vi "GUI_Bella_Laser.vi"() -> ()   [LabVIEW 2013]
uses:
  shared programs/GUI_Template/GUI_master/tcp_new_data_event.ctl
  shared programs/GUI_Template/GUI_master/tcp new data cluster.ctl
panel:
  out "XY Graph 8":cluster{dbl[], dbl[]}[](graph)
  out "XY Graph 7":cluster{dbl[], dbl[]}[](graph)
  in  "GUIdevice 4":string="LB_EnergyMeter_2"
  in  "GUIdevice 3":string="LB_EnergyMeter_1"
  in  "GUIdevice 2":string="RegenSpectrometer"
  out "FWHM::2":dbl caption="Regen FWHM" min=0.0 max=10000.0
  out "XY Graph 6":cluster{dbl[], dbl[]}[](graph)
  out "Thales.Spectrum_XPW_FWHM::1":dbl caption="Amp2 FWHM" min=-999.0 max=999999999.0
  out "Thales.Spectrum_Amp3_FWHM::1":dbl caption="Amp3 FWHM" min=-999.0 max=999999999.0
  out "Thales.Spectrum_Booster_FWHM::1":dbl caption="Booster FWHM" min=-999.0 max=999999999.0
  out "Thales.Spectrum_Preamp_FWHM::1":dbl caption="Amp1 FWHM" min=-999.0 max=999999999.0
  out "Thales.Spectrum_Regen_FWHM::1":dbl caption="Osc FWHM" min=-999.0 max=999999999.0
  out "XY Graph 5":cluster{dbl[], dbl[]}[](graph)
  in  "Clear":bool
  in  "GUIdevice 1":string="BellaTHALESsveECS"
  out "Reading.Channel 2::4":dbl caption="Amp3 (J)" min=0.0 max=0.0 format="%#.3f"
  out "Reading.Channel 2::3":dbl caption="Amp1 (mJ)" min=0.0 max=0.0
  out "Reading.Channel 1::4":dbl caption="Amp2 (J)" min=0.0 max=0.0 format="%#.3f"
  out "Reading.Channel 1::3":dbl caption="Preamp (mJ)" min=0.0 max=0.0
  out "tcp data event":T1
  in  "stop":bool
  out "error IO 2":errorcluster
  # "BELLA LASER STATS"
  # "Target"
  # "Target"
  # "Target"
  # "Target"
  # "Target"
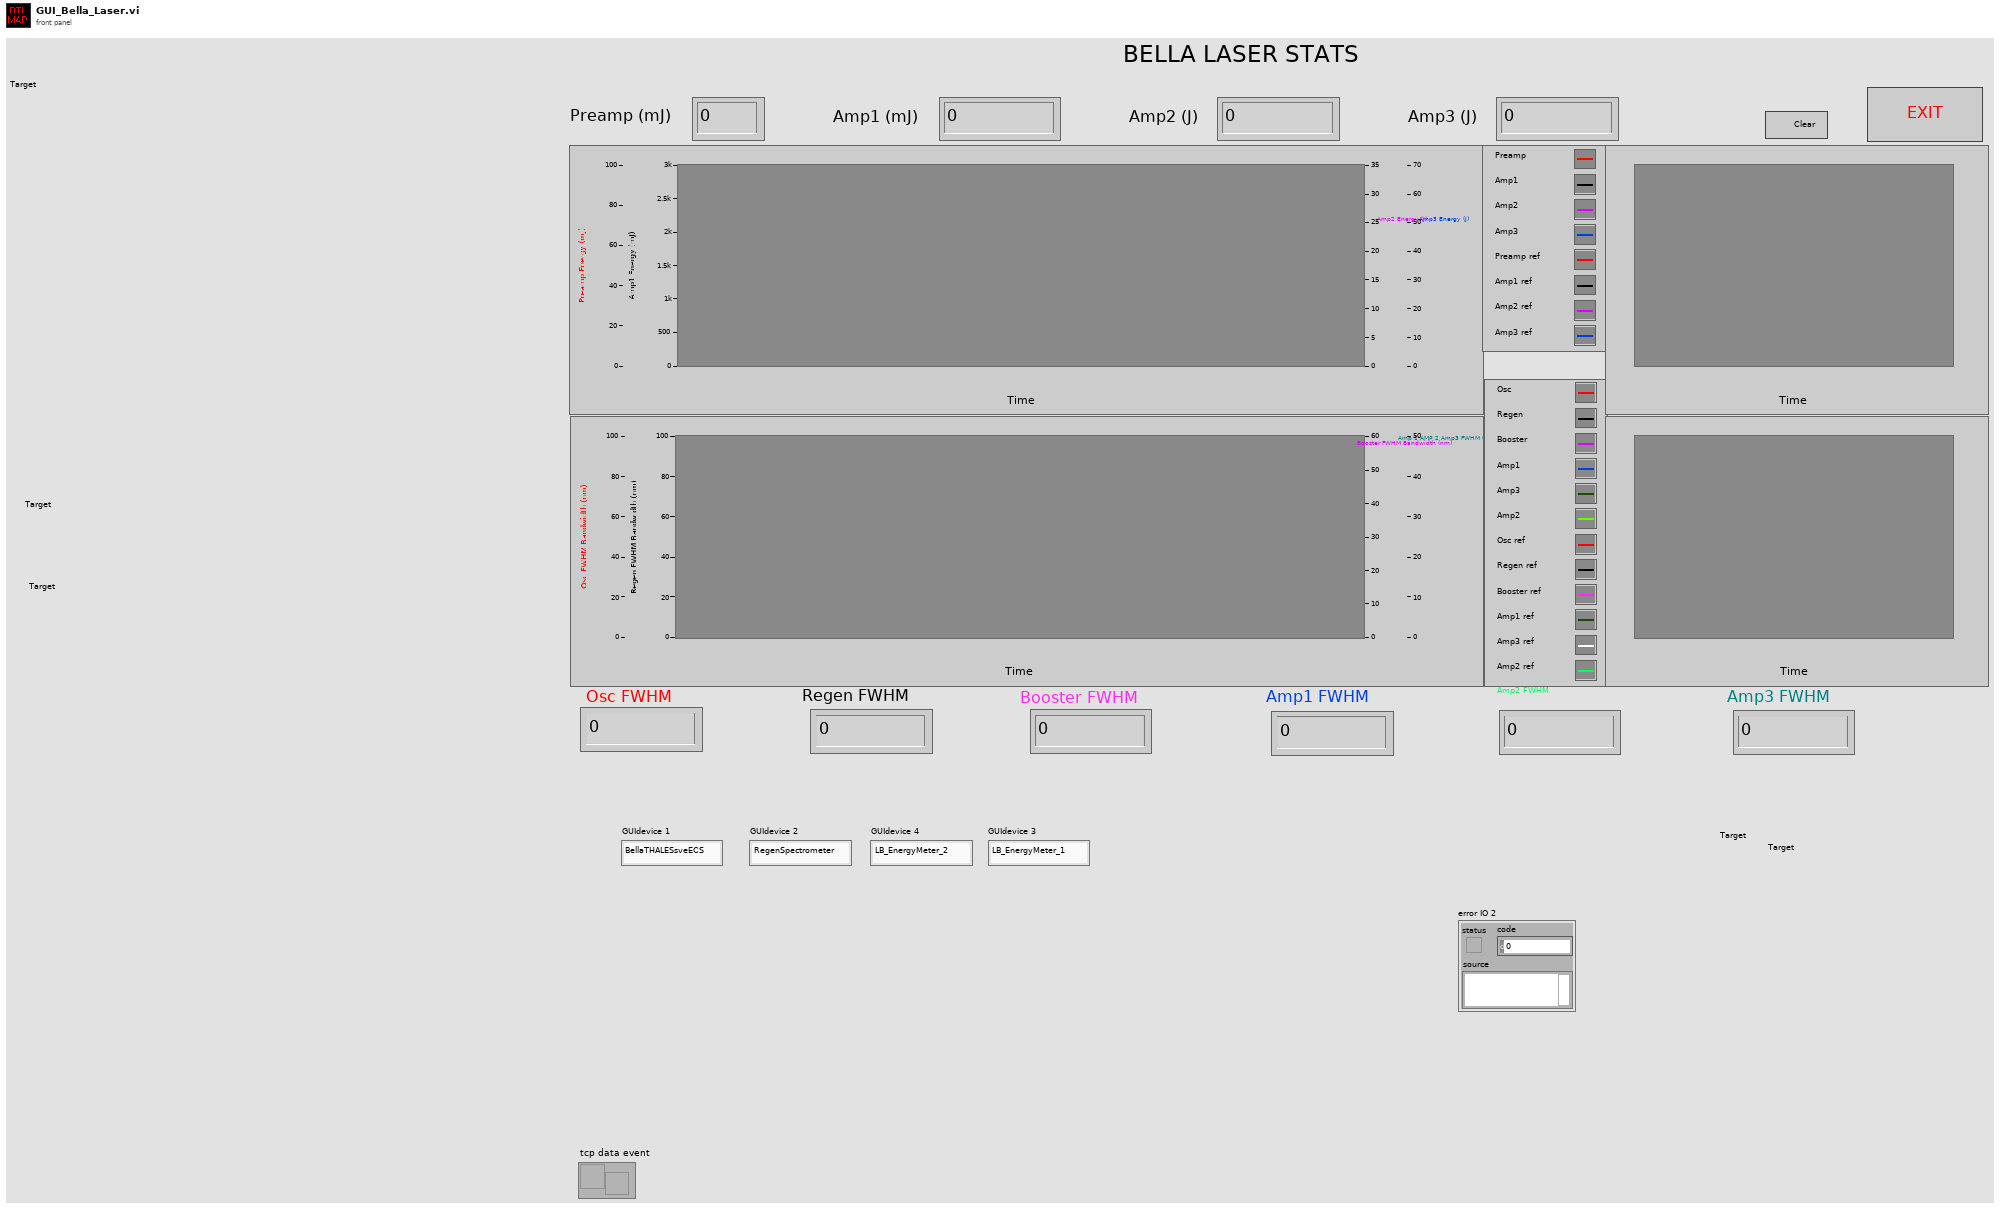
[diagram p1: front panel]
types:
  T1 = typedef "tcp_new_data_event.ctl" = refnum<user-event>
  T2 = typedef "tcp new data cluster.ctl" = cluster{"EventEnum":enum16{"new data", "connection status update"}, "Device name":string}
  T3 = cluster{"value 1":dbl, "value 2":dbl, "value 3":dbl, "value 4":dbl, "value 5":dbl, "ref 1":dbl, "ref 2":dbl, "ref 3":dbl, "ref 4":dbl, "ref 5":dbl, "value 6":dbl, "ref 6":dbl}
  T4 = cluster{"value 1":dbl, "value 2":dbl, "value 3":dbl, "value 4":dbl, "ref 1":dbl, "ref 2":dbl, "ref 3":dbl, "ref 4":dbl}
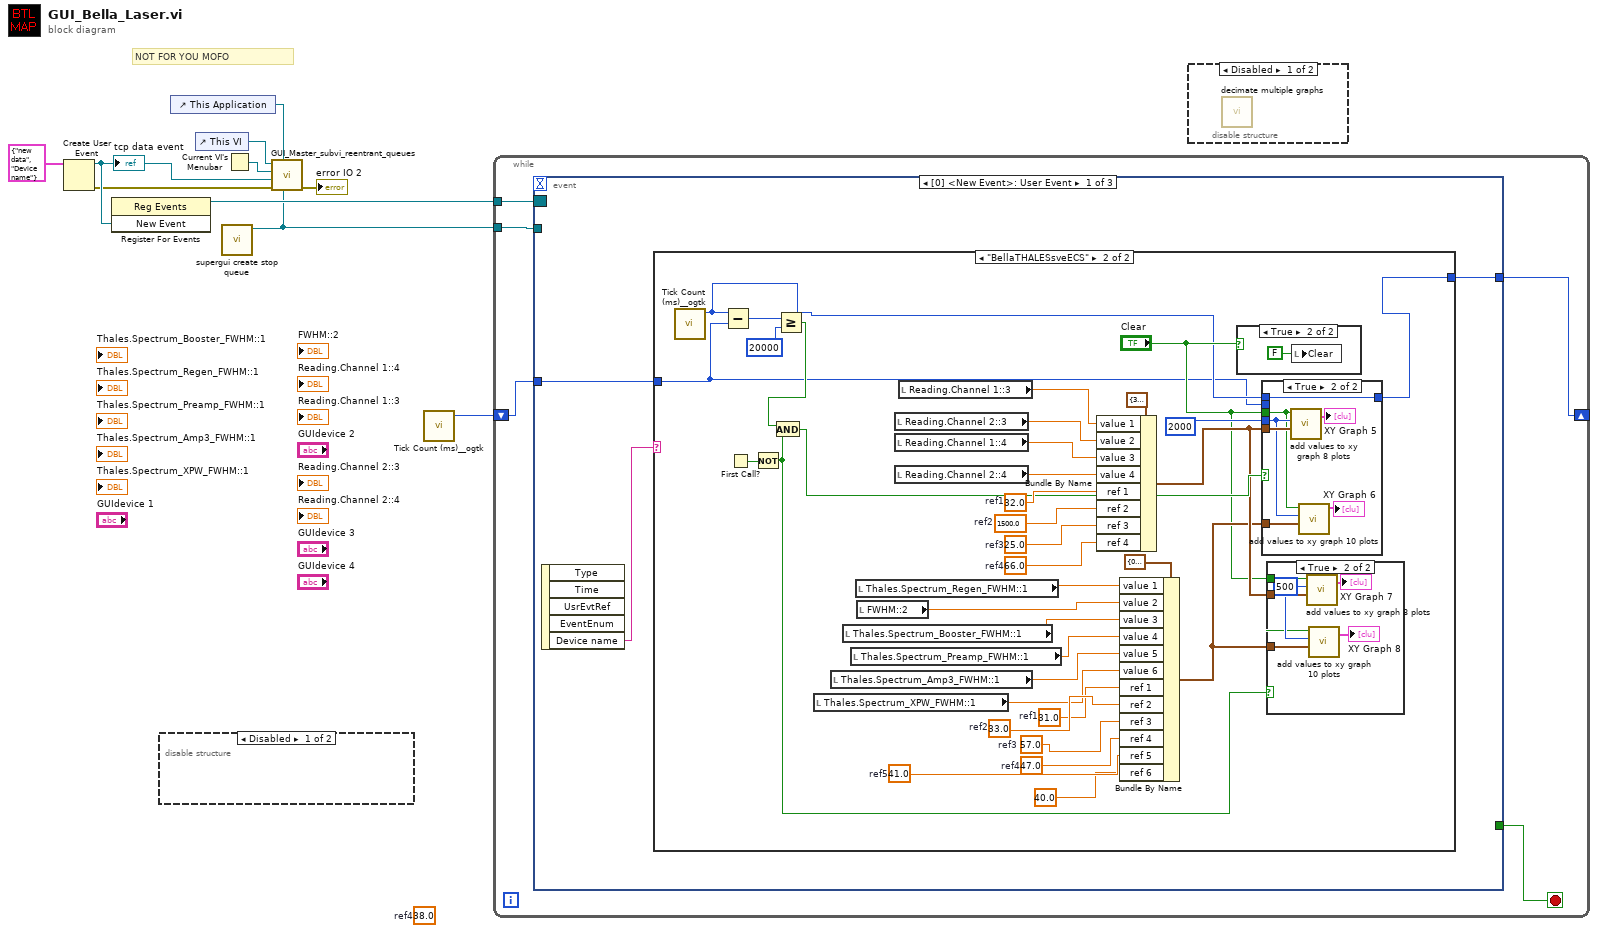
[diagram p0: block diagram]
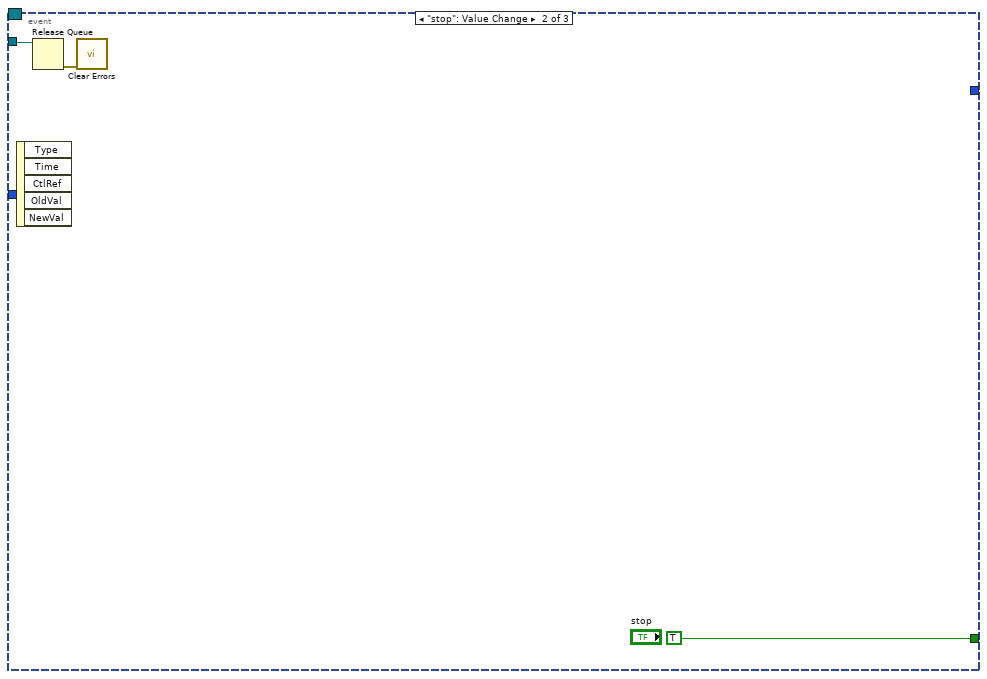
[diagram p8: hidden frame]
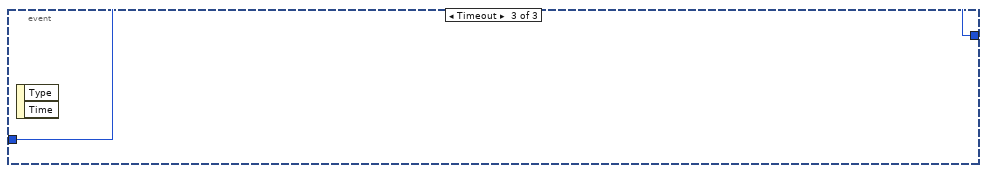
[diagram p9: hidden frame]
diagram:
  (unwired) 38.0  # ref4
  # "NOT FOR YOU MOFO"
  n1 = Create User Event(user event datatype=T2 {"EventEnum"=enum."new data", "Device name"="Device name"} ("New Event")) -> (user event=w9:refnum<user-event>, error out=w8:errorcluster)  [unwired: 1 in]
  "tcp data event" <- w9
  n2 = register-events(w9) -> (reference out=w4:refnum<event-registration>)  [unwired: 2 in, 1 out]
  n3 = disable-structure shown="Disabled" {
    frame Disabled {
    }
    frame Enabled {
    }
  }
  n4 = control-ref of="This Application"() -> (w10:refnum<vi>)
  n5 = control-ref of="This VI"() -> (w5:refnum<vi>)
  n6 = call "supergui create stop queue.vi"() -> ("STOP Queue out"=w1:refnum<queue>)  [unwired: 11 in]
  n7 = Current VI's Menubar() -> (w6:refnum<k9>)
  n8 = call "GUI_Master_subvi_reentrant_queues.vi"("STOP Queue in"=w1, "This Application"=w10, "error in (no error)"=w8, "tcp data event"=w9, "Caller menu reference"=w6, "Caller VI ref"=w5) -> ("error out"=→"error IO 2":errorcluster)  [unwired: 5 in]
  n9 = call <userlib>:"Tick Count (ms)__ogtk.vi"() -> ("millisecond timer value"=w2:u32)  [unwired: 10 in, 1 out]
  n10 = while {
    tunnel: w4 -> [w14]
    shift-right: [w12] -> _
    shift-left: w2 -> [w13]
    tunnel: w1 -> [w11]
    stop <- w15 stop-if-true
    n11 = event shown="[0] <New Event>: User Event" {
      selector: w14 -> [_ _ _]
      dyn-events: _ -> [_ _ _]
      timeout: _ -> [_ _ _]
      tunnel: [_ TRUE ("stop") _] -> w15
      tunnel: w13 -> [w17 _ w73]
      tunnel: [w16 _ w73] -> w12
      tunnel: w11 -> [_ w71 _]
      event User Event {
        n12 = event-data() -> ("Device name"=w18:string)  [unwired: 1 in, 4 out]
        n13 = case shown="\"BellaTHALESsveECS\"" w18 {
          tunnel: w17 -> [w19 w20]
          tunnel: [w19 w21] -> w16
          frame Default {
          }
          frame "BellaTHALESsveECS" {
            w32 = 41.0  # ref5
            w36 = 33.0  # ref2
            w34 = 47.0  # ref4
            w35 = 57.0  # ref3
            w33 = 31.0  # ref1
            w43 = 66.0  # ref4
            w44 = 25.0  # ref3
            w45 = 1500.0  # ref2
            w46 = 32.0  # ref1
            n14 = call <userlib>:"Tick Count (ms)__ogtk.vi"() -> ("millisecond timer value"=w22:u32)  [unwired: 10 in, 1 out]
            n15 = Subtract(x=w22, y=w20) -> (x-y=w53:u32)
            n16 = First Call?() -> (First Call?: T/F=w52:bool)
            n17 = Not(x=w52) -> (.not. x?=w23:bool)
            n18 = Greater Or Equal?(x=w53, y=u32 20000 ("min time between updates")) -> (x >= y?=w51:bool)
            n19 = And(x=w51, y=w23) -> (x .and. y?=w27:bool)
            n20 = local read "Thales.Spectrum_XPW_FWHM::1"() -> (w28:dbl)
            n21 = local read "Thales.Spectrum_Amp3_FWHM::1"() -> (w30:dbl)
            n22 = local read "Thales.Spectrum_Booster_FWHM::1"() -> (w38:dbl)
            n23 = local read "Thales.Spectrum_Preamp_FWHM::1"() -> (w37:dbl)
            n24 = local read "Thales.Spectrum_Regen_FWHM::1"() -> (w41:dbl)
            n25 = local read "FWHM::2"() -> (w39:dbl)
            n26 = local read "Reading.Channel 2::3"() -> (w49:dbl)
            n27 = local read "Reading.Channel 1::4"() -> (w48:dbl)
            n28 = local read "Reading.Channel 2::4"() -> (w47:dbl)
            n29 = local read "Reading.Channel 1::3"() -> (w50:dbl)
            n30 = Bundle By Name(cluster=T4 {"value 1"=32.0, "value 2"=32.0, "value 3"=32.0, "value 4"=32.0, "ref 1"=32.0, "ref 2"=32.0, "ref 3"=32.0, "ref 4"=32.0} ("inputs"), "value 1"=w50, "value 2"=w49, "value 3"=w48, "value 4"=w47, "ref 1"=w46, "ref 2"=w45, "ref 3"=w44, "ref 4"=w43) -> (w26:T4)
            n31 = Bundle By Name(cluster=T3 {"value 1"=0.0, "value 2"=0.0, "value 3"=0.0, "value 4"=0.0, "value 5"=0.0, "ref 1"=0.0, "ref 2"=0.0, "ref 3"=0.0, "ref 4"=0.0, "ref 5"=0.0, "value 6"=0.0, "ref 6"=0.0} ("inputs"), "value 1"=w41, "value 2"=w39, "value 3"=w38, "value 4"=w37, "value 5"=w30, "value 6"=w28, "ref 1"=w33, "ref 2"=w36, "ref 3"=w35, "ref 4"=w34, "ref 5"=w32, "ref 6"=40.0) -> (w25:T3)
            n32 = case shown="True" "Clear" {
              frame False {
              }
              frame True {
                n33 = local write "Clear"(FALSE ("Clear")) -> ()
              }
            }
            n34 = case shown="True" w27 {
              tunnel: w26 -> [_ w68]
              tunnel: 2000 ("max # data points") -> [_ w67]
              tunnel: "Clear" -> [_ w66]
              tunnel: w25 -> [_ w65]
              tunnel: w22 -> [_ w62]
              tunnel: [w61 w62] -> w21
              tunnel: w20 -> [w61 _]
              frame False {
              }
              frame True {
                n35 = call "add values to xy graph 8 plots.vi"("inputs"=w68, "max # points"=w67, "Clear"=w66) -> ("xy graph"=→"XY Graph 5":cluster{dbl[], dbl[]}[])  [unwired: 8 in]
                n36 = call "add values to xy graph 10 plots.vi"("inputs"=w65, "max # points"=w67, "Clear"=w66) -> ("xy graph"=→"XY Graph 6":cluster{dbl[], dbl[]}[])  [unwired: 8 in]
              }
            }
            n37 = case shown="True" w23 {
              tunnel: w26 -> [_ w59]
              tunnel: w25 -> [_ w58]
              tunnel: "Clear" -> [_ w56]
              frame False {
              }
              frame True {
                w57 = 500 ("max # points")
                n38 = call "add values to xy graph 8 plots.vi"("inputs"=w59, "max # points"=w57, "Clear"=w56) -> ("xy graph"=→"XY Graph 7":cluster{dbl[], dbl[]}[])  [unwired: 8 in]
                n39 = call "add values to xy graph 10 plots.vi"("inputs"=w58, "max # points"=w57, "Clear"=w56) -> ("xy graph"=→"XY Graph 8":cluster{dbl[], dbl[]}[])  [unwired: 8 in]
              }
            }
          }
        }
      }
      event "stop": Value Change {
        n40 = event-data() -> ()  [unwired: 1 in, 5 out]
        n41 = Release Queue(queue=w71) -> (error out=w70:errorcluster)  [unwired: 2 in, 2 out]
        n42 = call <vilib>:"Clear Errors.vi"("error in (no error)"=w70) -> ()  [unwired: 6 in, 1 out]
      }
      event Timeout {
        n43 = event-data() -> ()  [unwired: 1 in, 2 out]
      }
    }
  }
  n44 = disable-structure shown="Disabled" {
    frame Disabled {
      n45 = call "decimate multiple graphs.vi"() -> ()  [unwired: 11 in, 1 out]
    }
    frame Enabled {
    }
  }
